vi "Image Color Table.vi"() -> ()   [LabVIEW 2016]
uses:
  graph_utilities.lvclass
panel:
  in  "Custom Colors []":u32[](array[colorbox])=[10420479, 16860, 3381759, 6618880, 16772608, 16711680]
  in  "CET":T1(ring)
  in  "Test Image":enum16{"Bitches Brew", "Color Map"}(ring)
  in  "Color Map":T2(ring)
  out "Image":u32[][](graph)
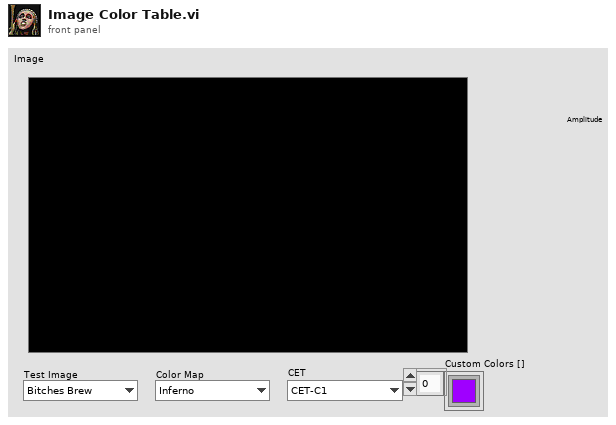
[diagram p1: front panel]
types:
  T1 = enum16{"CET-C1", "CET-C1s", "CET-C2", "CET-C2s", "CET-C3", "CET-C3s", "CET-C4", "CET-C4s", "CET-C5", "CET-C5s", "CET-C6", "CET-C6s", "CET-C7", "CET-C7s", "CET-CBC1", "CET-CBC2", "CET-CBD1", "CET-CBL1", "CET-CBL2", "CET-D01", "CET-D01A", "CET-D02", "CET-D03", "CET-D04", "CET-D06", "CET-D07", "CET-D08", "CET-D09", "CET-D10", "CET-D11", "CET-D12", "CET-D13", "CET-I1", "CET-I2", "CET-I3", "CET-L01", "CET-L02", "CET-L03", "CET-L04", "CET-L05", "CET-L06", "CET-L07", "CET-L08", "CET-L09", "CET-L10", "CET-L11", "CET-L12", "CET-L13", "CET-L14", "CET-L15", "CET-L16", "CET-L17", "CET-L18", "CET-L19", "CET-L20", "CET-R1", "CET-R2", "CET-R3", "CET-R4"}
  T2 = enum16{"Inferno", "Kindlmann", "Plasma", "Viridis", "LevyLab2010", "ColorCET...", "Custom..."}
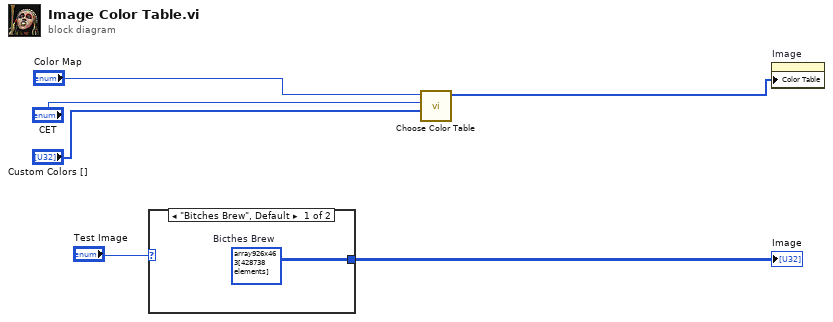
[diagram p0: block diagram]
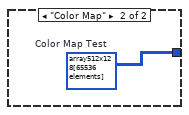
[diagram p2: hidden frame]
diagram:
  n1 = case shown="\"Bitches Brew\", Default" "Test Image" {
    tunnel: [w7 w8] -> w5
    frame "Bitches Brew", Default {
      w7 = u32[][] array926x463[428738 elements]  # Bicthes Brew
    }
    frame "Color Map" {
      w8 = u32[][] array512x128[65536 elements]  # Color Map Test
    }
  }
  "Image" <- w5
  n2 = call "Choose Color Table.vi"("Custom Table"="Custom Colors []", "ColorCET"="CET", "Color Map"="Color Map") -> ("Color Table"=w4:u32[])  [unwired: 5 in, 3 out]
  n3 = property on="Image" class="IntGraph (strict)"("Color Table"=w4) -> ()  [unwired: 2 in, 2 out]
